vi "Parameter Setting.vi"(11 "TEST INFO":T2) -> (3 "IN 2":T1)   [LabVIEW 2013]
panel:
  in  "OK Button":bool
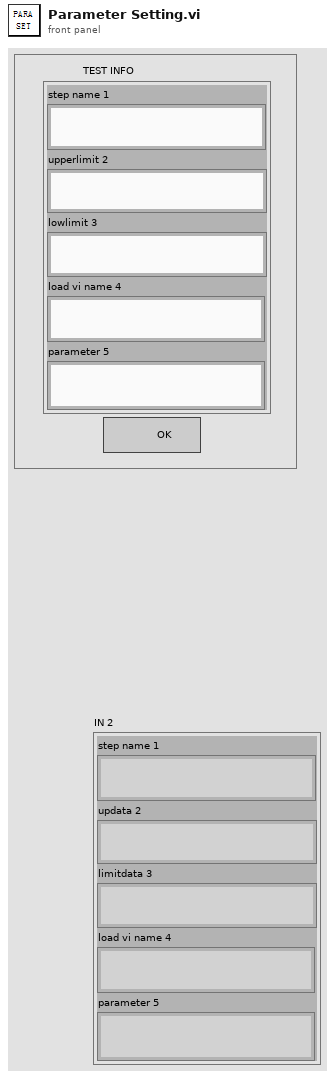
[diagram p1: front panel]
types:
  T1 = cluster{"step name 1":string, "updata 2":string, "limitdata 3":string, "load vi name 4":string, "parameter 5":string}
  T2 = cluster{"step name 1":string, "upperlimit 2":string, "lowlimit 3":string, "load vi name 4":string, "parameter 5":string}
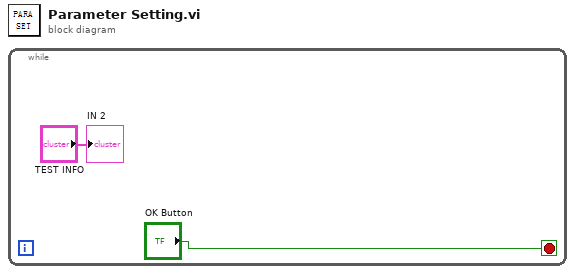
[diagram p0: block diagram]
diagram:
  n1 = while {
    stop <- "OK Button" stop-if-true
    "IN 2" <- "TEST INFO"
  }
